vi "Frame Rate Control (SubVI).vi"(11 "Replay Frame Rate":u32=10) -> ()   [LabVIEW 2015]
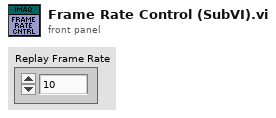
[diagram p1: front panel]
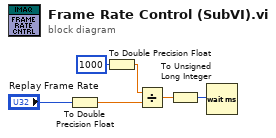
[diagram p0: block diagram]
diagram:
  n1 = To Double Precision Float(number="Replay Frame Rate") -> (double precision float=w6:dbl)
  n2 = To Double Precision Float(number=u32 1000 ("x")) -> (double precision float=w5:dbl)
  n3 = Divide(x=w5, y=w6) -> (x/y=w1:dbl)
  n4 = To Unsigned Long Integer(number=w1) -> (unsigned 32bit integer=w4:u32)
  n5 = Wait (ms)(milliseconds to wait=w4) -> ()  [unwired: 1 out]
